vi "ObjectNotification.vi"() -> ()   [LabVIEW 2010]
uses:
  EDSDK-Labview.llb/kEdsObjectEvents.ctl
  kernel32.dll
panel:
  out "handler pointer":u32
  out "notifier":u32
  out "event":u32
  out "firing":bool
  in  "inRef":u32=4294967295
  in  "object":bool
  in  "fire":bool
  in  "stop":bool
  out "ref":u32
  out "Time":u32
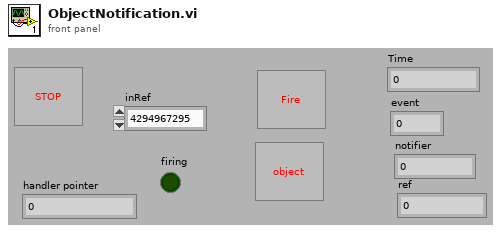
[diagram p1: front panel]
types:
  T1 = typedef "kEdsObjectEvents.ctl" = u32
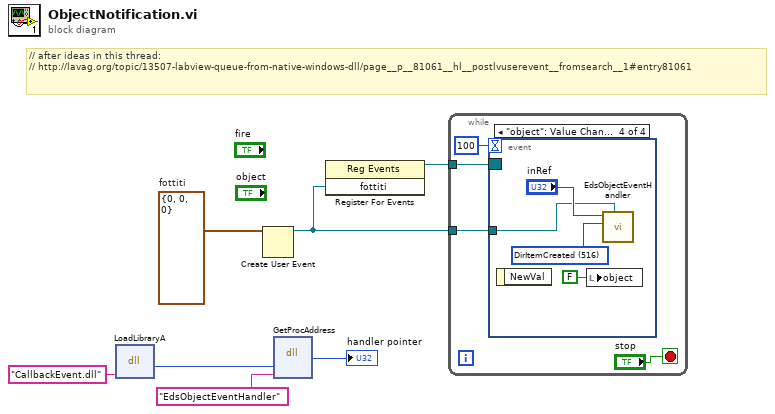
[diagram p0: block diagram]
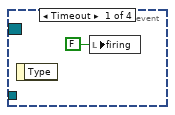
[diagram p2: hidden frame]
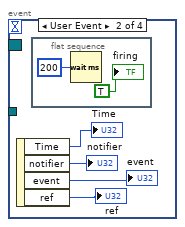
[diagram p3: hidden frame]
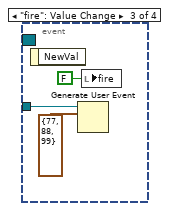
[diagram p4: hidden frame]
diagram:
  w5 = cluster{"notifier":u32, "event":u32, "ref":u32} {"notifier"=0, "event"=0, "ref"=0}  # fottiti
  # "// after ideas in this thread:\n// http://lavag.org/topic/13507-labview-queue-from-native-windows-dll/page__p__81061__hl__postlvuserevent__fromsearch__1#entry81061"
  n1 = dll-call lib="kernel32.dll" fn="LoadLibraryA"("libraryName"="CallbackEvent.dll") -> ("return type"=w3:u32)  [unwired: 4 in, 2 out]
  n2 = Create User Event(user event datatype=w5) -> (user event=w6:refnum<user-event>)  [unwired: 1 in, 1 out]
  n3 = dll-call lib="kernel32.dll" fn="GetProcAddress"("address"=w3, "procName"="EdsObjectEventHandler") -> ("return type"=→"handler pointer":u32)  [unwired: 5 in, 2 out]
  n4 = register-events(w6) -> (reference out=w7:refnum<event-registration>)  [unwired: 2 in, 1 out]
  n5 = while {
    tunnel: w6 -> [w9]
    tunnel: w7 -> [w8]
    stop <- "stop" stop-if-true
    n6 = event shown="[3] \"object\": Value Change" {
      selector: w8 -> [_ _ _ _]
      dyn-events: _ -> [_ _ _ _]
      timeout: 100 -> [_ _ _ _]
      tunnel: w9 -> [_ _ w20 w22]
      event Timeout {
        n7 = event-data() -> ()  [unwired: 1 in, 1 out]
        n8 = local write "firing"(FALSE ("firing")) -> ()
      }
      event User Event {
        n9 = event-data() -> ("Time"=→"Time":u32, "notifier"=→"notifier":u32, "event"=→"event":u32, "ref"=→"ref":u32)  [unwired: 1 in]
        n10 = flat-sequence {
          frame #0 {
            n11 = Wait (ms)(milliseconds to wait=u32 200) -> ()  [unwired: 1 out]
            "firing" <- TRUE ("firing")
          }
        }
      }
      event "fire": Value Change {
        n12 = event-data() -> ()  [unwired: 1 in, 1 out]
        n13 = Generate User Event(user event=w20, event data cluster=cluster{"notifier":i32, "event":i32, "ref":i32} {"notifier"=77, "event"=88, "ref"=99}) -> ()  [unwired: 1 in, 2 out]
        n14 = local write "fire"(FALSE ("fire")) -> ()
      }
      event "object": Value Change {
        w24 = T1 516 items=["All"=512, "VolumeInfoChanged"=513, "VolumeUpdateItems"=514, "FolderUpdateItems"=515, "DirItemCreated"=516, "DirItemRemoved"=517, "DirItemInfoChanged"=518, "DirItemContentChanged"=519, "DirItemRequestTransfer"=520, "DirItemRequestTransferDT"=521, "DirItemCancelTransferDT"=522, "VolumeAdded"=524, "VolumeRemoved"=525] ("inEvent")
        n15 = event-data() -> ()  [unwired: 1 in, 1 out]
        n16 = local write "object"(FALSE ("object")) -> ()
        n17 = call "EdsObjectEventHandler.vi"("LV user event"=w22, "inEvent"=w24, "inRef"="inRef") -> ()  [unwired: 4 in, 2 out]
      }
    }
  }
